vi "idg_trust_persuader.vi"(9 "Inverted":bool, 10 "Input Diagnostic State":T1, 11 "output":dbl) -> (3 "output out":dbl)   [LabVIEW 2011]
uses:
  idg_trust_t.ctl
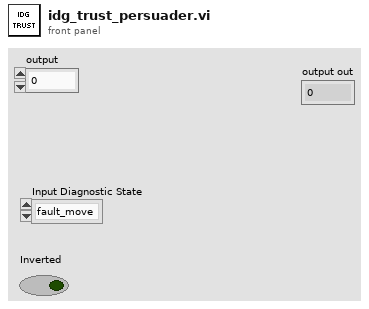
[diagram p1: front panel]
types:
  T1 = typedef "idg_trust_t.ctl" = enum16{"fault_move", "fault_high", "fault_low", "out_high", "out_low", "trust"}
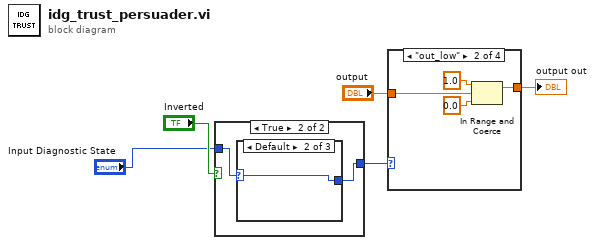
[diagram p0: block diagram]
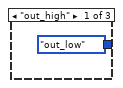
[diagram p3: hidden frame]
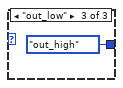
[diagram p4: hidden frame]
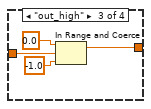
[diagram p6: hidden frame]
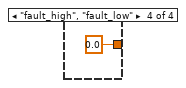
[diagram p7: hidden frame]
diagram:
  n1 = case shown="True" "Inverted" {
    tunnel: "Input Diagnostic State" -> [w6 w8]
    tunnel: [w6 w7] -> w1
    frame False {
    }
    frame True {
      n2 = case shown="Default" w8 {
        selector: w8 -> [_ w10 _]
        tunnel: [idg_trust_t."out_low" ("Input Diagnostic State") w10 idg_trust_t."out_high" ("Input Diagnostic State")] -> w7
        frame "out_high" {
        }
        frame Default {
        }
        frame "out_low" {
        }
      }
    }
  }
  n3 = case shown="\"out_low\"" w1 {
    tunnel: "output" -> [w12 w16 w20 _]
    tunnel: [w12 w15 w19 0.0 ("upper limit")] -> w4
    frame "trust", Default {
    }
    frame "out_low" {
      n4 = In Range and Coerce(upper limit=1.0, x=w16, lower limit=0.0) -> (coerced(x)=w15:dbl)  [unwired: 1 out]
    }
    frame "out_high" {
      n5 = In Range and Coerce(upper limit=0.0, x=w20, lower limit=-1.0) -> (coerced(x)=w19:dbl)  [unwired: 1 out]
    }
    frame "fault_high", "fault_low" {
    }
  }
  "output out" <- w4
